vi "Configure Serial Channel Tap Display Parameters.vi"(0 "fpga interface in":refnum<k20>, 5 "serial channel configurations":T1[](array[typedef]) {"RAW Display Parameters"."Bayer Parameters"."Blue Gain" format="%_4g"; "RAW Display Parameters"."Bayer Parameters"."Green Gain" format="%_4g"; "RAW Display Parameters"."Bayer Parameters"."Red Gain" format="%_4g"; "RAW Display Parameters"."Bayer Parameters"."Algorithm" items=["Bilinear", "VNG"]; "RAW Display Parameters"."Bayer Parameters"."Pattern" items=["GB", "GR", "BG", "RG"]}, 11 "error in (no error)":errorcluster) -> (4 "fpga interface out":refnum<k20>, 6 "serial channel display parameters":T6[](array[typedef]) {"RAW parameters"."bayer parameters"."blue gain" format="%_4g"; "RAW parameters"."bayer parameters"."green gain" format="%_4g"; "RAW parameters"."bayer parameters"."red gain" format="%_4g"; "RAW parameters"."bayer parameters"."algorithm" items=["Bilinear", "VNG"]; "RAW parameters"."bayer parameters"."pattern" items=["GB", "GR", "BG", "RG"]}, 8 "serial input channels":string[](array[string]), 10 "serial output channels":string[](array[string]), 15 "error out":errorcluster)   [LabVIEW 2023, in "GettingStarted_Tap_148X_Host.lvlib"]
uses:
  GettingStarted_Tap_148X_Host.lvlib
  Common/Types/Serial Channel Display Parameters.ctl
  <vilib>/vision/Image Controls.llb/IMAQ Image.ctl
  Common/Types/RAW Interpretation for Display.ctl
  Types/Serial Channel Tap Configuration.ctl
  Types/Serial Channel Tap Pair.ctl
  <instrlib>/FlexRIO/CSI-2/v2/FPGA/Types/Display Parameters.ctl
  <instrlib>/FlexRIO/CSI-2/v2/Common/Types/LLP Data Type.ctl
  Common/Types/Serial Channel Configuration.ctl
  Common/GettingStarted_Common_148X_Host.lvlib
  <instrlib>/FlexRIO/CSI-2/v2/Common/NI CSI-2 API Common v2.lvlib
  <instrlib>/FlexRIO/CSI-2/v2/FPGA/NI CSI-2 API FPGA v2.lvlib
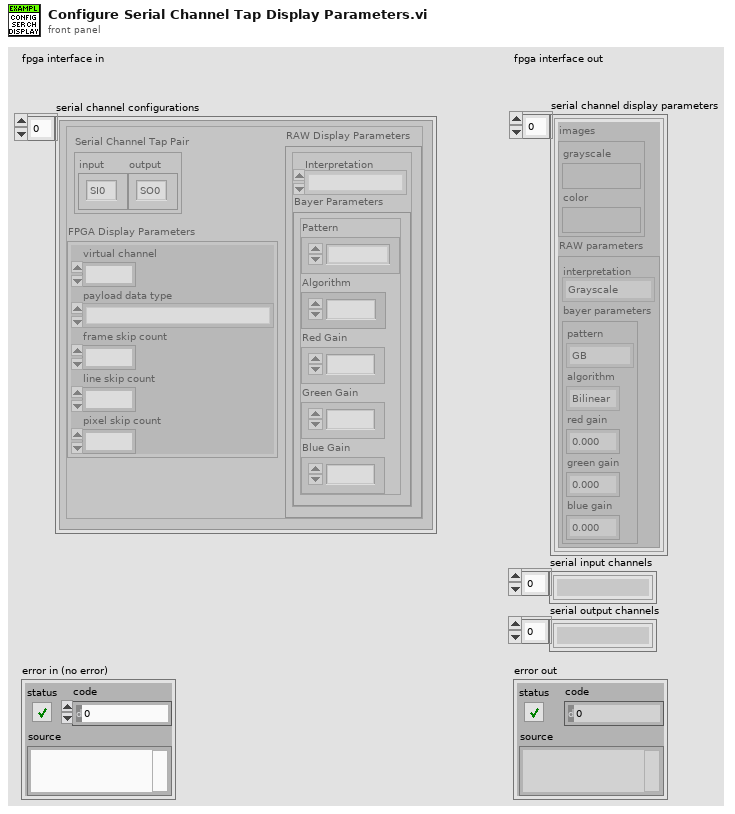
[diagram p1: front panel]
types:
  T1 = typedef "GettingStarted_Tap_148X_Host.lvlib/Serial Channel Tap Configuration.ctl" = cluster{"Serial Channel Tap Pair":T2, "FPGA Display Parameters":T3, "RAW Display Parameters":cluster{"Interpretation":T5, "Bayer Parameters":cluster{"Pattern":i32, "Algorithm":i32, "Red Gain":dbl, "Green Gain":dbl, "Blue Gain":dbl}}}
  T2 = typedef "GettingStarted_Tap_148X_Host.lvlib/Serial Channel Tap Pair.ctl" = cluster{"input":string, "output":string}
  T3 = typedef "NI CSI-2 API FPGA v2.lvlib/Display Parameters.ctl" = cluster{"virtual channel":fxp<+,4,4>, "payload data type":T4, "frame skip count":u16, "line skip count":u8, "pixel skip count":fxp<+,5,5>}
  T4 = typedef "NI CSI-2 API Common v2.lvlib/LLP Data Type.ctl" = enum8{"Frame Start", "Frame End", "Line Start", "Line End", "End of Transmission", "Reserved 0", "Reserved 1", "Reserved 2", "Generic Short Packet 1", "Generic Short Packet 2", "Generic Short Packet 3", "Generic Short Packet 4", "Generic Short Packet 5", "Generic Short Packet 6", "Generic Short Packet 7", "Generic Short Packet 8", "Null", "Blanking Data", "Embedded 8-bit non Image Data", "Generic Long Packet 1", "Generic Long Packet 2", "Generic Long Packet 3", "Generic Long Packet 4", "Reserved 3", "YUV420 8-bit", "YUV420 10-bit", "Legacy YUV420 8-bit", "Reserved 4", "YUV420 8-bit Chroma Shifted", "YUV420 10-bit Chroma Shifted", "YUV422 8-bit", "YUV422 10-bit", "RGB444", "RGB555", "RGB565", "RGB666", "RGB888", "Reserved 5", "Reserved 6", "RAW 24", "RAW 6", "RAW 7", "RAW 8", "RAW 10", "RAW 12", "RAW 14", "RAW 16", "RAW 20", "User Defined 8-bit Data 1", "User Defined 8-bit Data 2", "User Defined 8-bit Data 3", "User Defined 8-bit Data 4", "User Defined 8-bit Data 5", "User Defined 8-bit Data 6", "User Defined 8-bit Data 7", "User Defined 8-bit Data 8", "USL Command", "Reserved 7", "Reserved 8", "Reserved 9", "Reserved 10", "Reserved 11", "Reserved 12", "LRTE EPD Spacer"}
  T5 = typedef "GettingStarted_Common_148X_Host.lvlib/RAW Interpretation for Display.ctl" = enum16{"Grayscale", "Bayer", "RGB", "YUV422", "YUV420", "Legacy YUV420"}
  T6 = typedef "GettingStarted_Common_148X_Host.lvlib/Serial Channel Display Parameters.ctl" = cluster{"images":cluster{"grayscale":T7, "color":T7}, "RAW parameters":cluster{"interpretation":T5, "bayer parameters":cluster{"pattern":i32, "algorithm":i32, "red gain":dbl, "green gain":dbl, "blue gain":dbl}}}
  T7 = typedef "IMAQ Image.ctl" = refnum<image>
  T8 = typedef "GettingStarted_Common_148X_Host.lvlib/Serial Channel Configuration.ctl" = cluster{"Serial Channel":string, "FPGA Display Parameters":T3, "RAW Display Parameters":cluster{"Interpretation":T5, "Bayer Parameters":cluster{"Pattern":i32, "Algorithm":i32, "Red Gain":dbl, "Green Gain":dbl, "Blue Gain":dbl}}}
  T9 = cluster{"Interpretation":T5, "Bayer Parameters":cluster{"Pattern":i32, "Algorithm":i32, "Red Gain":dbl, "Green Gain":dbl, "Blue Gain":dbl}}
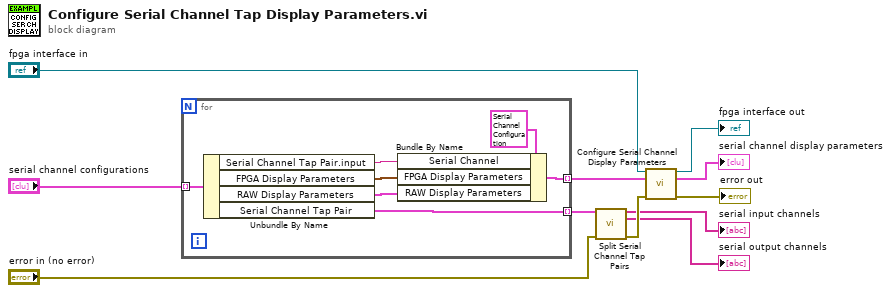
[diagram p0: block diagram]
diagram:
  n1 = for {
    tunnel: "serial channel configurations" -> [w18] mode=indexing
    tunnel: [w17] -> w10 mode=indexing
    tunnel: [w13] -> w8 mode=indexing
    n2 = Unbundle By Name(w18) -> ("Serial Channel Tap Pair.input"=w15:string, "FPGA Display Parameters"=w14:T3, "RAW Display Parameters"=w12:T9, "Serial Channel Tap Pair"=w17:T2)
    n3 = Bundle By Name(cluster=T8 {"Serial Channel"="", "FPGA Display Parameters"={"virtual channel"=0.0, "payload data type"=enum."Frame Start", "frame skip count"=0, "line skip count"=0, "pixel skip count"=0.0}, "RAW Display Parameters"={"Interpretation"=enum."Grayscale", "Bayer Parameters"={"Pattern"=0, "Algorithm"=0, "Red Gain"=0.0, "Green Gain"=0.0, "Blue Gain"=0.0}}} ("Channel Configuration"), "Serial Channel"=w15, "FPGA Display Parameters"=w14, "RAW Display Parameters"=w12) -> (w13:T8)
  }
  n4 = call "Split Serial Channel Tap Pairs.vi"("serial channel tap pairs"=w10, "error in (no error)"="error in (no error)") -> ("serial input channels"=→"serial input channels":string[], "serial output channels"=→"serial output channels":string[], "error out"=w6:errorcluster)  [unwired: 11 in]
  n5 = call "Configure Serial Channel Display Parameters.vi"("fpga interface in"="fpga interface in", "serial channel configurations"=w8, "error in (no error)"=w6) -> ("fpga interface out"=→"fpga interface out":refnum<k20>, "serial channel display parameters"=→"serial channel display parameters":T6[], "error out"=→"error out":errorcluster)  [unwired: 9 in, 1 out]
